vi "CreateUint16.vi"(10 "high":u8, 11 "low":u8) -> (3 "Numeric 3":u16)   [LabVIEW 2016]
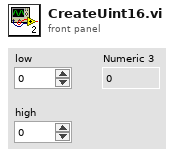
[diagram p1: front panel]
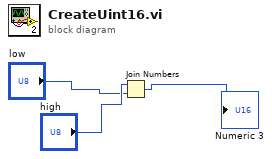
[diagram p0: block diagram]
diagram:
  n1 = Join Numbers(hi="high", lo="low") -> ((hi.lo)=→"Numeric 3":u16)
